vi "add project items.vi"(7 "top level library":string, 8 "error in (no error)":errorcluster, 9 "items to add":string[](array[string]), 10 "Project in":refnum<vi>, 11 "NI_AB_API_PPL in":refnum<class "NI_AB_API_PPL.lvclass">) -> (0 "error out":errorcluster, 3 "NI_AB_API_PPL out":refnum<class "NI_AB_API_PPL.lvclass">)   [LabVIEW 2024]
doc: "Add items to the project and configures the build specification directory"
uses:
  <vilib>/AppBuilder/AB_API/PPL/NI_AB_API_PPL.lvclass
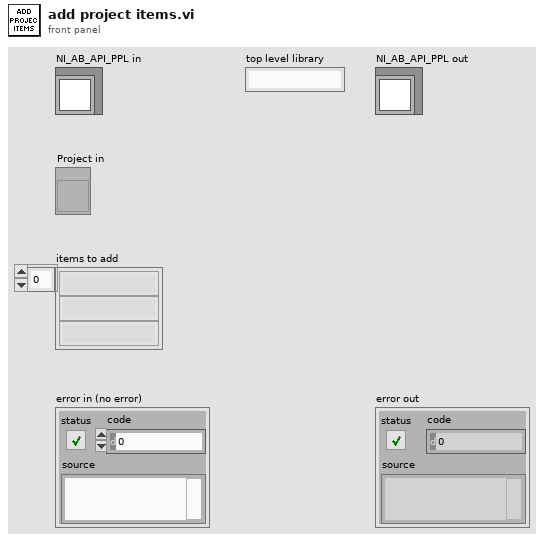
[diagram p1: front panel]
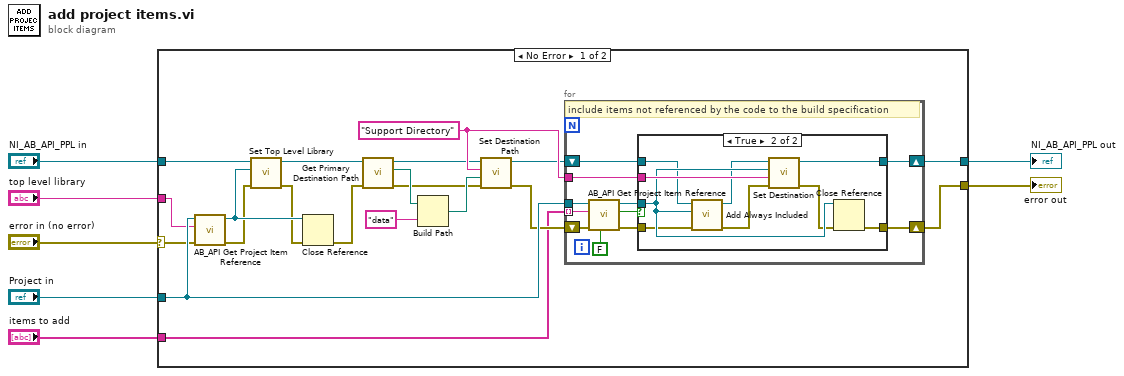
[diagram p0: block diagram]
diagram:
  n1 = case shown="No Error" "error in (no error)" {
    selector: "error in (no error)" -> [w25 w51]
    tunnel: "Project in" -> [w27 _]
    tunnel: "NI_AB_API_PPL in" -> [w26 w50]
    tunnel: [w22 w51] -> w4
    tunnel: [w21 w50] -> w3
    tunnel: "items to add" -> [w12 _]
    tunnel: "top level library" -> [w8 _]
    frame No Error {
      w23 = "Support Directory" ("Destination label")
      n2 = call <vilib>:"AB_API Get Project Item Reference.vi"("error in (no error)"=w25, "Name"=w8, "Project Refnum"=w27) -> ("error out"=w9:errorcluster, "ProjectItem Refnum"=w11:refnum<vi>)  [unwired: 6 in, 1 out]
      n3 = call-dynamic "Set Top Level Library.vi"("error in (no error)"=w9, "ProjectItem Refnum"=w11, "PPL in"=w26) -> ("error out"=w10:errorcluster, "PPL out"=w13:refnum<class "NI_AB_API_PPL.lvclass">)  [unwired: 7 in]
      n4 = Close Reference(reference=w11, error in (no error)=w10) -> (error out=w14:errorcluster)
      n5 = call-dynamic "Get Primary Destination Path.vi"("error in (no error)"=w14, "PPL in"=w13) -> ("error out"=w18:errorcluster, "Primary destination path"=w19:path, "PPL out"=w17:refnum<class "NI_AB_API_PPL.lvclass">)  [unwired: 7 in]
      n6 = Build Path(base path=w19, name or relative path="data" ("Destination label")) -> (appended path=w20:path)
      n7 = call-dynamic "Set Destination Path.vi"("error in (no error)"=w18, "Destination path"=w20, "Destination label"=w23, "PPL in"=w17) -> ("error out"=w15:errorcluster, "PPL out"=w16:refnum<class "NI_AB_API_PPL.lvclass">)  [unwired: 6 in]
      n8 = for {
        tunnel: w27 -> [w34]
        tunnel: w12 -> [w33] mode=indexing
        shift-right: [w35] -> w22
        shift-left: w15 -> [w38]
        shift-right: [w36] -> w21
        shift-left: w16 -> [w32]
        tunnel: w23 -> [w28]
        # "include items not referenced by the code to the build specification"
        n9 = call <vilib>:"AB_API Get Project Item Reference.vi"("Exclude dependencies"=FALSE, "error in (no error)"=w38, "Name"=w33, "Project Refnum"=w34) -> ("error out"=w37:errorcluster, "found?"=w30:bool, "ProjectItem Refnum"=w31:refnum<vi>)  [unwired: 5 in]
        n10 = case shown="True" w30 {
          tunnel: w37 -> [w39 w41]
          tunnel: [w40 w42] -> w36
          tunnel: [w39 w49] -> w35
          tunnel: w32 -> [w40 w45]
          tunnel: w31 -> [_ w47]
          tunnel: w28 -> [_ w48]
          frame False {
          }
          frame True {
            n11 = call-dynamic "Add Always Included.vi"("error in (no error)"=w41, "ProjectItem Refnum"=w47, "PPL in"=w45) -> ("error out"=w44:errorcluster, "PPL out"=w46:refnum<class "NI_AB_API_PPL.lvclass">)  [unwired: 7 in]
            n12 = call-dynamic "Set Destination.vi"("error in (no error)"=w44, "Destination label"=w48, "ProjectItem Refnum"=w47, "DLL in"=w46) -> ("error out"=w43:errorcluster, "DLL out"=w42:refnum<class "NI_AB_API_PPL.lvclass">)  [unwired: 6 in]
            n13 = Close Reference(reference=w47, error in (no error)=w43) -> (error out=w49:errorcluster)
          }
        }
      }
    }
    frame Error {
    }
  }
  "error out" <- w4
  "NI_AB_API_PPL out" <- w3
